vi "RH200 CONTROLLER w RH meter.vi"() -> ()   [LabVIEW 2014]
uses:
  <vilib>/Instr/_visa.llb/VISA Configure Serial Port (Instr).vi
  <vilib>/Utility/file.llb/Write To Spreadsheet File (string).vi
  <vilib>/Utility/file.llb/Read From Spreadsheet File (string).vi
  <vilib>/DAQmx/write.llb/DAQmx Write (Analog DBL 1Chan 1Samp).vi
  <vilib>/DAQmx/write.llb/DAQmx Write (Digital Bool 1Line 1Point).vi
  <vilib>/DAQmx/read.llb/DAQmx Read (Analog DBL 1Chan 1Samp).vi
panel:
  out "File path":path
  out "Exhaust temp (C)":dbl
  out "Exhaust RH (%)":dbl
  out "error out":errorcluster
  out "sequence preview":cluster{"Array":dbl[], "Array":dbl[]}[](graph)
  out "Current step":i32
  in  "Delay between data points (s)":dbl=2.0 caption="Wet MFC (V)" format="%#_13g"
  in  "stop when\nsequence\nends":bool=TRUE
  in  "Save data during sequence":bool=TRUE
  in  "Log data":bool
  out "Saving data":bool
  in  "stop":bool
  out "Sequence end time":string
  in  "Run sequence":bool
  in  "Import sequence file":bool
  in  "Save sequence":bool
  in  "Clear sequence":bool
  in  "Sequence control":string[][](table)
  in  "Set RH (%)":dbl=2.0 min=2.0 max=90.0 step=1.0
  in  "enable generator":bool
  in  "clear chart":bool
  out "Waveform Chart":cluster{"RH Setpoint":dbl, "RH":dbl}(graph)
  in  "Temp":dbl=25.0 caption="Temp (C)" format="%#_13g"
  # "User sequence"
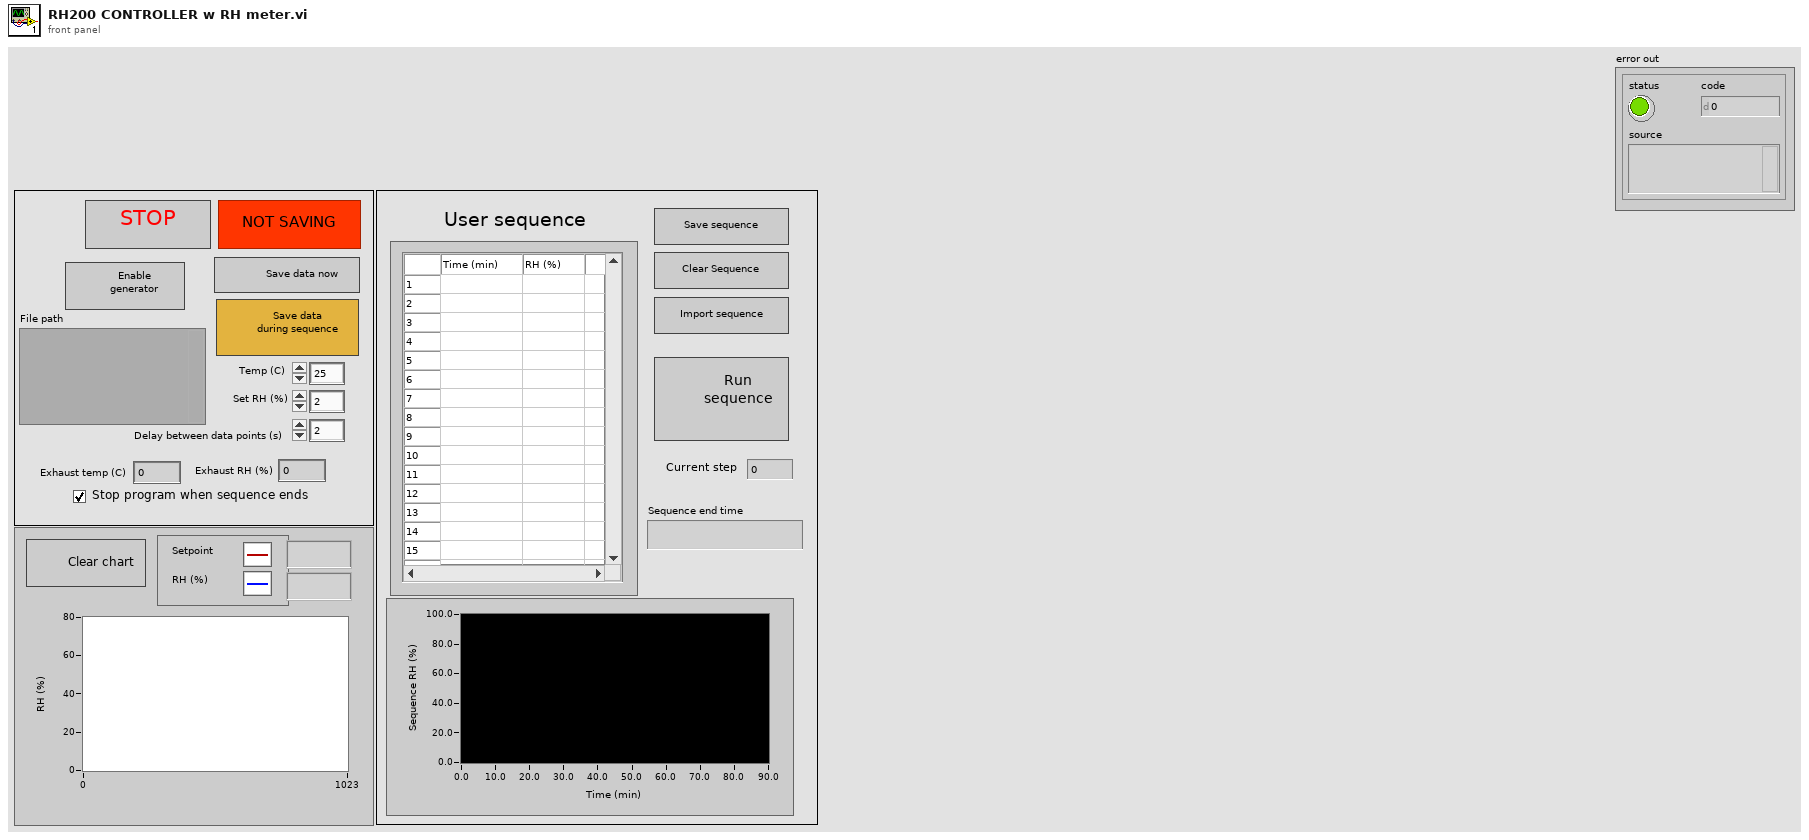
[diagram p1: front panel]
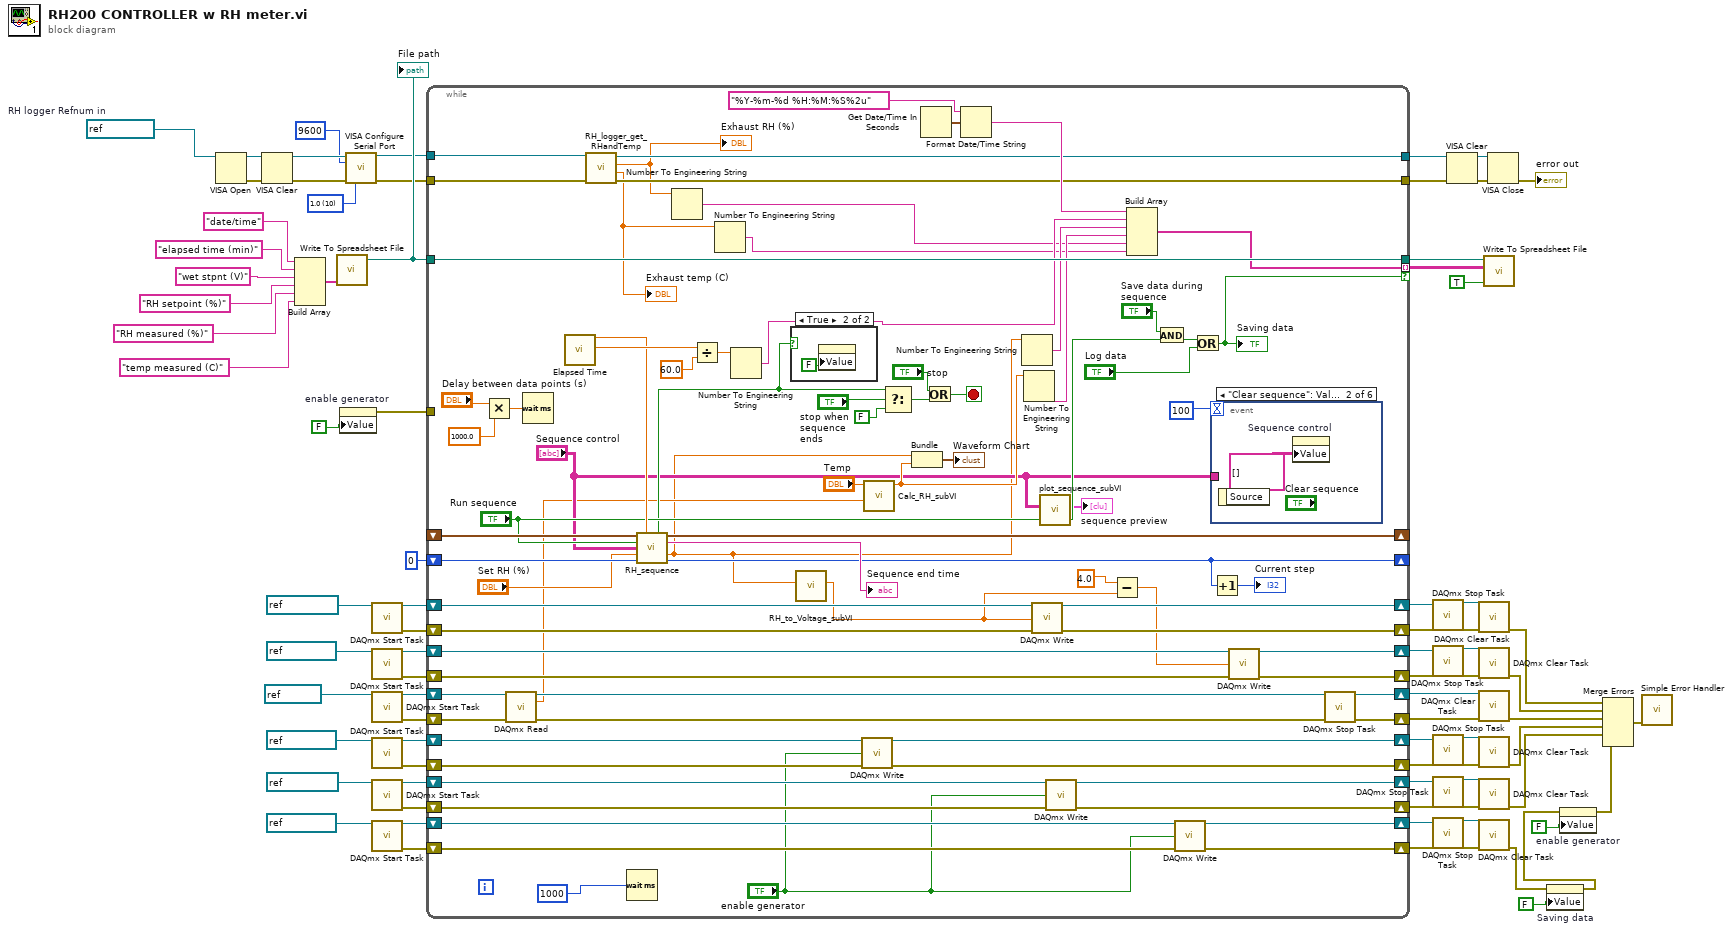
[diagram p0: block diagram]
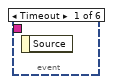
[diagram p3: hidden frame]
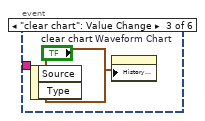
[diagram p4: hidden frame]
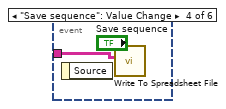
[diagram p5: hidden frame]
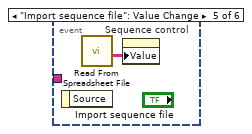
[diagram p6: hidden frame]
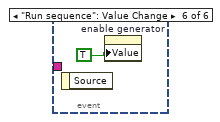
[diagram p7: hidden frame]
diagram:
  w10 = refnum<visa-resource-name> "COM15"  # RH logger Refnum in
  w12 = u16 10 items=["1.0"=10, "1.5"=15, "2.0"=20] ("stop bits (10: 1 bit)")
  n1 = VISA Open(VISA resource name=w10) -> (VISA resource name=w9:refnum<visa-resource-name>, error out=w8:errorcluster)  [unwired: 4 in]
  n2 = VISA Clear(VISA resource name=w9, error in (no error)=w8) -> (VISA resource name out=w14:refnum<visa-resource-name>, error out=w13:errorcluster)
  n3 = Build Array("date/time" ("time format string (%c)"), "elapsed time (min)" ("time format string (%c)"), "wet stpnt (V)" ("time format string (%c)"), "RH setpoint (%)" ("time format string (%c)"), "RH measured (%)" ("time format string (%c)"), "temp measured (C)" ("time format string (%c)")) -> (w29:string[])
  n4 = call-poly <vilib>:"Write To Spreadsheet File.vi"("1D data"=w29) -> ("new file path (Not A Path if cancelled)"=w31:path)  [unwired: 7 in]
  "File path" <- w31
  n5 = property on="enable generator" class="Bool (strict)"("Value"=FALSE ("enable generator")) -> (error out=w21:errorcluster)  [unwired: 2 in, 1 out]
  n6 = call-poly "VISA Configure Serial Port"("VISA resource name"=w14, "baud rate (9600)"=u32 9600, "error in (no error)"=w13, "stop bits (10: 1 bit)"=w12) -> ("VISA resource name out"=w7:refnum<visa-resource-name>, "error out"=w6:errorcluster)  [unwired: 10 in]
  n7 = call <vilib>:"DAQmx Start Task.vi"("task/channels in"=refnum<k21> "AO WET") -> ("task out"=w45:refnum<k21>, "error out"=w46:errorcluster)  [unwired: 13 in]
  n8 = call <vilib>:"DAQmx Start Task.vi"("task/channels in"=refnum<k21> "AO DRY") -> ("task out"=w48:refnum<k21>, "error out"=w47:errorcluster)  [unwired: 13 in]
  n9 = call <vilib>:"DAQmx Start Task.vi"("task/channels in"=refnum<k21> "AI DP") -> ("task out"=w78:refnum<k21>, "error out"=w77:errorcluster)  [unwired: 13 in]
  n10 = call <vilib>:"DAQmx Start Task.vi"("task/channels in"=refnum<k21> "DO DRY") -> ("task out"=w73:refnum<k21>, "error out"=w74:errorcluster)  [unwired: 13 in]
  n11 = call <vilib>:"DAQmx Start Task.vi"("task/channels in"=refnum<k21> "DO WET") -> ("task out"=w62:refnum<k21>, "error out"=w61:errorcluster)  [unwired: 13 in]
  n12 = call <vilib>:"DAQmx Start Task.vi"("task/channels in"=refnum<k21> "DO GAS") -> ("task out"=w59:refnum<k21>, "error out"=w60:errorcluster)  [unwired: 13 in]
  n13 = while {
    shift-right: [w152] -> w76
    shift-left: w78 -> [w159]
    shift-right: [w151] -> w75
    shift-left: w77 -> [w158]
    shift-right: [w148] -> w71
    shift-left: w73 -> [w149]
    shift-right: [w147] -> w68
    shift-left: w74 -> [w150]
    shift-right: [w145] -> w64
    shift-left: w62 -> [w144]
    shift-right: [w146] -> w67
    shift-left: w61 -> [w143]
    shift-right: [w140] -> w57
    shift-left: w59 -> [w141]
    shift-right: [w139] -> w54
    shift-left: w60 -> [w142]
    shift-right: [w137] -> w50
    shift-left: w48 -> [w136]
    shift-right: [w138] -> w53
    shift-left: w47 -> [w135]
    shift-right: [w132] -> w43
    shift-left: w45 -> [w133]
    shift-right: [w131] -> w40
    shift-left: w46 -> [w134]
    tunnel: [w130] -> w32
    tunnel: w31 -> [w130]
    tunnel: [w122] -> w27 mode=indexing if=w104
    shift-right: [w97] -> _
    shift-left: 0 ("current step out") -> [w121]
    shift-right: [w119] -> _
    shift-left: _ -> [w120]
    tunnel: w21 -> [_]
    tunnel: w7 -> [w87]
    tunnel: w6 -> [w86]
    tunnel: [w85] -> w5
    tunnel: [w84] -> w4
    stop <- w99 stop-if-true
    n14 = Multiply(x="Delay between data points (s)", y=1000.0) -> (x*y=w100:dbl)
    n15 = call-poly <vilib>:"DAQmx Read.vi"("task/channels in"=w159, "error in"=w158) -> ("task out"=w154:refnum<k21>, "data"=w90:dbl, "error out"=w153:errorcluster)  [unwired: 11 in]
    n16 = Wait (ms)(milliseconds to wait=w100) -> ()  [unwired: 1 out]
    n17 = call "Elapsed Time"() -> ("Present (s)"=w116:dbl, "Elapsed Time (s)"=w129:dbl)  [unwired: 12 in, 6 out]
    n18 = call "RH_logger_get_RHandTemp.vi"("error in (no error)"=w86, "VISA resource name"=w87) -> ("error out"=w84:errorcluster, "Temp (C)"=w82:dbl, "RH (%)"=w83:dbl, "VISA resource name out"=w85:refnum<visa-resource-name>)  [unwired: 6 in]
    "Exhaust RH (%)" <- w83
    "Exhaust temp (C)" <- w82
    n19 = Wait (ms)(milliseconds to wait=u32 1000) -> ()  [unwired: 1 out]
    n20 = call "RH_sequence.vi"("present second in"=w120, "present second"=w116, "run sequence"="Run sequence", "Sequence control"="Sequence control", "set RH"="Set RH (%)", "current step in"=w121) -> ("sequence done?"=w103:bool, "present second out"=w119:timestamp, "Sequence end time"=→"Sequence end time":string, "set RH 2"=w89:dbl, "current step out"=w97:i32)  [unwired: 3 in, 2 out]
    n21 = Number To Engineering String ("elapsed time (min)")(4:w83) -> (0:w81:string)  [unwired: 3 in]
    n22 = Divide(x=w129, y=60.0) -> (x/y=w124:dbl)
    n23 = Number To Engineering String ("elapsed time (min)")(4:w82) -> (0:w80:string)  [unwired: 3 in]
    n24 = Number To Engineering String ("elapsed time (min)")(4:w124) -> (0:w123:string)  [unwired: 3 in]
    n25 = case shown="True" w103 {
      frame False {
      }
      frame True {
        n26 = property on="Run sequence" class="Bool (strict)"("Value"=FALSE ("Run sequence")) -> ()  [unwired: 2 in, 2 out]
      }
    }
    n27 = call "RH_to_Voltage_subVI.vi"("RH"=w89) -> ("set point (V)"=w88:dbl)  [unwired: 10 in]
    n28 = call-poly <vilib>:"DAQmx Write.vi"("task/channels in"=w149, "data"="enable generator", "error in"=w150) -> ("task out"=w148:refnum<k21>, "error out"=w147:errorcluster)  [unwired: 10 in, 1 out]
    n29 = call "Calc_RH_subVI.vi"("DP"=w90, "Temp"="Temp") -> ("RH"=w114:dbl)  [unwired: 9 in]
    n30 = Select(t=w103, s="stop when\nsequence\nends", f=FALSE) -> (s? t:f=w109:bool)
    n31 = Bundle("set RH 2"=w89, "RH"=w114) -> (→"Waveform Chart":cluster{"set RH 2":dbl, "RH":dbl})  [unwired: 1 in]
    n32 = Get Date/Time In Seconds() -> (seconds since 1Jan1904=w127:timestamp)
    n33 = Or(x="stop", y=w109) -> (x .or. y?=w99:bool)
    n34 = Format Date/Time String(time format string (%c)="%Y-%m-%d %H:%M:%S%2u", seconds (now)=w127) -> (date/time string=w125:string)  [unwired: 1 in]
    n35 = Number To Engineering String ("elapsed time (min)")(4:w89) -> (0:w115:string)  [unwired: 3 in]
    n36 = Number To Engineering String ("elapsed time (min)")(4:w114) -> (0:w113:string)  [unwired: 3 in]
    n37 = call-poly <vilib>:"DAQmx Write.vi"("task/channels in"=w133, "data"=w88, "error in"=w134) -> ("task out"=w132:refnum<k21>, "error out"=w131:errorcluster)  [unwired: 10 in, 1 out]
    n38 = call "plot_sequence_subVI.vi"("User-defined sequence"="Sequence control") -> ("Array"=→"sequence preview":cluster{"Array":dbl[], "Array":dbl[]}[])  [unwired: 10 in]
    n39 = call-poly <vilib>:"DAQmx Write.vi"("task/channels in"=w144, "data"="enable generator", "error in"=w143) -> ("task out"=w145:refnum<k21>, "error out"=w146:errorcluster)  [unwired: 10 in, 1 out]
    n40 = Subtract(x=4.0 ("data"), y=w88) -> (x-y=w94:dbl)
    n41 = Build Array(w125, w123, w115, w113, w81, w80) -> (w122:string[])
    n42 = And(x="Save data during sequence", y="Run sequence") -> (x .and. y?=w106:bool)
    n43 = call-poly <vilib>:"DAQmx Write.vi"("task/channels in"=w141, "data"="enable generator", "error in"=w142) -> ("task out"=w140:refnum<k21>, "error out"=w139:errorcluster)  [unwired: 10 in, 1 out]
    n44 = Or(x=w106, y="Log data") -> (x .or. y?=w104:bool)
    "Saving data" <- w104
    n45 = event shown="[1] \"Clear sequence\": Value Change" {
      selector: _ -> [_ _ _ _ _ _]
      dyn-events: _ -> [_ _ _ _ _ _]
      timeout: 100 -> [_ _ _ _ _ _]
      tunnel: "Sequence control" -> [_ _ _ w163 _ _]
      event Timeout {
        n46 = event-data() -> ()  [unwired: 1 in, 1 out]
      }
      event "Clear sequence": Value Change {
        n47 = event-data() -> ()  [unwired: 1 in, 1 out]
        n48 = property on="Sequence control" class="Tbl (strict)"("Value"=string[][] []) -> ()  [unwired: 2 in, 2 out]
      }
      event "clear chart": Value Change {
        n49 = event-data() -> ()  [unwired: 1 in, 2 out]
        n50 = property on="Waveform Chart" class="WFChart (strict)"("History Data"=cluster{"RH Setpoint":dbl, "RH":dbl}[] []) -> ()  [unwired: 2 in, 2 out]
      }
      event "Save sequence": Value Change {
        n51 = event-data() -> ()  [unwired: 1 in, 1 out]
        n52 = call-poly <vilib>:"Write To Spreadsheet File.vi"("2D data"=w163) -> ()  [unwired: 7 in, 1 out]
      }
      event "Import sequence file": Value Change {
        n53 = event-data() -> ()  [unwired: 1 in, 1 out]
        n54 = call-poly <vilib>:"Read From Spreadsheet File.vi"() -> ("all rows"=w164:string[][])  [unwired: 7 in, 4 out]
        n55 = property on="Sequence control" class="Tbl (strict)"("Value"=w164) -> ()  [unwired: 2 in, 2 out]
      }
      event "Run sequence": Value Change {
        n56 = event-data() -> ()  [unwired: 1 in, 1 out]
        n57 = property on="enable generator" class="Bool (strict)"("Value"=TRUE ("enable generator")) -> ()  [unwired: 2 in, 2 out]
      }
    }
    n58 = Increment(x=w97) -> (x+1=→"Current step":i32)
    n59 = call-poly <vilib>:"DAQmx Write.vi"("task/channels in"=w136, "data"=w94, "error in"=w135) -> ("task out"=w137:refnum<k21>, "error out"=w138:errorcluster)  [unwired: 10 in, 1 out]
    n60 = call <vilib>:"DAQmx Stop Task.vi"("task/channels in"=w154, "error in"=w153) -> ("task out"=w152:refnum<k21>, "error out"=w151:errorcluster)  [unwired: 12 in]
  }
  n61 = call <vilib>:"DAQmx Stop Task.vi"("task/channels in"=w43, "error in"=w40) -> ("task out"=w42:refnum<k21>, "error out"=w41:errorcluster)  [unwired: 12 in]
  n62 = call <vilib>:"DAQmx Stop Task.vi"("task/channels in"=w50, "error in"=w53) -> ("task out"=w51:refnum<k21>, "error out"=w52:errorcluster)  [unwired: 12 in]
  n63 = call <vilib>:"DAQmx Stop Task.vi"("task/channels in"=w71, "error in"=w68) -> ("task out"=w70:refnum<k21>, "error out"=w69:errorcluster)  [unwired: 12 in]
  n64 = call <vilib>:"DAQmx Stop Task.vi"("task/channels in"=w64, "error in"=w67) -> ("task out"=w65:refnum<k21>, "error out"=w66:errorcluster)  [unwired: 12 in]
  n65 = call <vilib>:"DAQmx Stop Task.vi"("task/channels in"=w57, "error in"=w54) -> ("task out"=w56:refnum<k21>, "error out"=w55:errorcluster)  [unwired: 12 in]
  n66 = VISA Clear(VISA resource name=w5, error in (no error)=w4) -> (VISA resource name out=w17:refnum<visa-resource-name>, error out=w16:errorcluster)
  n67 = call <vilib>:"DAQmx Clear Task.vi"("task in"=w42, "error in"=w41) -> ("error out"=w39:errorcluster)  [unwired: 13 in]
  n68 = call <vilib>:"DAQmx Clear Task.vi"("task in"=w51, "error in"=w52) -> ("error out"=w38:errorcluster)  [unwired: 13 in]
  n69 = call <vilib>:"DAQmx Clear Task.vi"("task in"=w76, "error in"=w75) -> ("error out"=w36:errorcluster)  [unwired: 13 in]
  n70 = call <vilib>:"DAQmx Clear Task.vi"("task in"=w70, "error in"=w69) -> ("error out"=w35:errorcluster)  [unwired: 13 in]
  n71 = call <vilib>:"DAQmx Clear Task.vi"("task in"=w65, "error in"=w66) -> ("error out"=w34:errorcluster)  [unwired: 13 in]
  n72 = call <vilib>:"DAQmx Clear Task.vi"("task in"=w56, "error in"=w55) -> ("error out"=w23:errorcluster)  [unwired: 13 in]
  n73 = call-poly <vilib>:"Write To Spreadsheet File.vi"("append to file? (new file:F)"=TRUE, "2D data"=w27, "file path (dialog if empty)"=w32) -> ()  [unwired: 5 in, 1 out]
  n74 = VISA Close(VISA resource name=w17, error in (no error)=w16) -> (error out=→"error out":errorcluster)
  n75 = property on="Saving data" class="Bool (strict)"(error in=w23, "Value"=FALSE ("enable generator")) -> (error out=w19:errorcluster)  [unwired: 1 in, 1 out]
  n76 = property on="enable generator" class="Bool (strict)"(error in=w19, "Value"=FALSE ("enable generator")) -> (error out=w18:errorcluster)  [unwired: 1 in, 1 out]
  n77 = Merge Errors(w39, w38, w36, w35, w34, w18) -> (w37:errorcluster)
  n78 = call <vilib>:"Simple Error Handler.vi"("error in (no error)"=w37) -> ()  [unwired: 4 in, 5 out]
